vi "Add Response (Result from Request).vi"(7 "Request":refnum<class "Request.lvclass">, 8 "error in (no error)":errorcluster, 10 "JSON Value in":variant, 11 "Server in":refnum<class "JSONRPC Server.lvclass">) -> (0 "error out":errorcluster, 1 "response string":string, 3 "Server out":refnum<class "JSONRPC Server.lvclass">)   [LabVIEW 2020, in "JSON-RPC Lib.lvlib" / "JSONRPC Server.lvclass"]
uses:
  JSONRPC Server.lvclass
  Request/Request.lvclass
  Request/Request.lvclass/Request.ctl
  Request/request.Read jsonrpc.vi
  Request/request.Read id value.vi
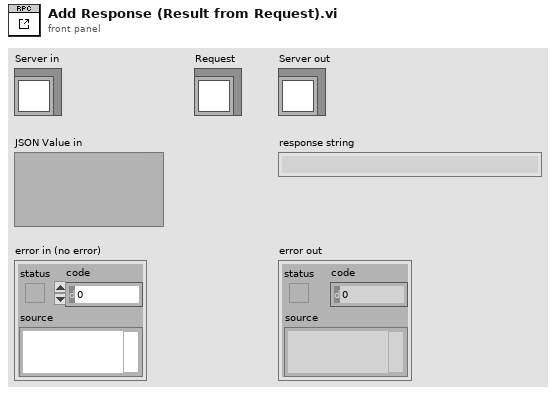
[diagram p1: front panel]
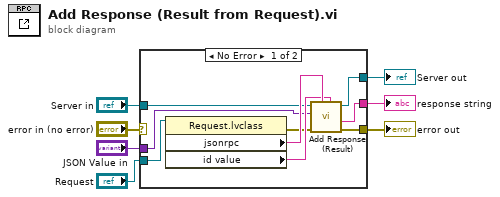
[diagram p0: block diagram]
diagram:
  n1 = case shown="No Error" "error in (no error)" {
    selector: "error in (no error)" -> [_ w18]
    tunnel: [w11 w18] -> w4
    tunnel: [w9 w17] -> w5
    tunnel: "Server in" -> [w10 w17]
    tunnel: "Request" -> [w16 _]
    tunnel: "JSON Value in" -> [w13 _]
    tunnel: [w8 _] -> w1
    frame No Error {
      n2 = property class="Request.lvclass"(reference=w16) -> (error out=w12:errorcluster, "jsonrpc"=w15:string, "id value"=w14:string)  [unwired: 1 in, 1 out]
      n3 = call "Add Response (Result).vi"("id value"=w14, "jsonrpc"=w15, "error in (no error)"=w12, "JSON Value in"=w13, "Server in"=w10) -> ("error out"=w11:errorcluster, "response string"=w8:string, "Server out"=w9:refnum<class "JSONRPC Server.lvclass">)  [unwired: 4 in]
    }
    frame Error {
    }
  }
  "error out" <- w4
  "Server out" <- w5
  "response string" <- w1
